vi "numberToString.vi"(8 "error in (no error)":errorcluster, 10 "Numeric":dbl, 11 "ScriptEvent in":refnum<class "ScriptEvent.lvclass">) -> (0 "error out":errorcluster, 2 "String":string, 3 "ScriptEvent out":refnum<class "ScriptEvent.lvclass">)   [LabVIEW 2009, in "Tools.lvlib" / "Scripting.lvlib" / "ScriptEvent.lvclass"]
uses:
  ScriptEvent.lvclass
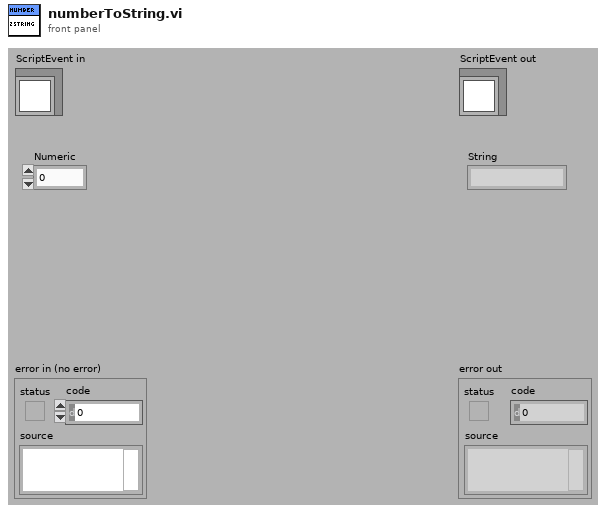
[diagram p1: front panel]
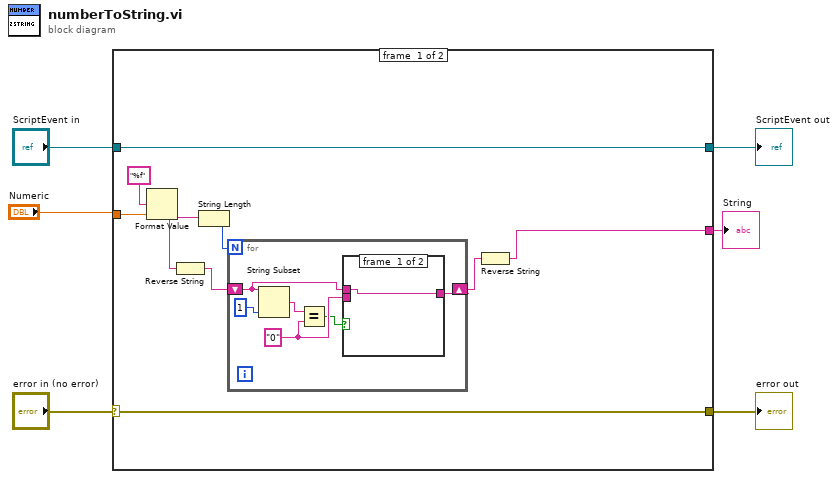
[diagram p0: block diagram]
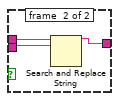
[diagram p2: hidden frame]
diagram:
  n1 = case shown="No Error" "error in (no error)" {
    selector: "error in (no error)" -> [w14 w27]
    tunnel: [w14 w27] -> w2
    tunnel: [w15 w26] -> w3
    tunnel: "ScriptEvent in" -> [w15 w26]
    tunnel: "Numeric" -> [w8 _]
    tunnel: [w7 _] -> w1
    frame #0 {
      n2 = Format Value(format string="%f", value (0)=w8) -> (output string=w9:string)  [unwired: 1 in]
      n3 = Reverse String(1:w9) -> (0:w12:string)
      n4 = String Length(string=w9) -> (length=w11:i32)
      n5 = for {
        N: w11 -> [_]
        shift-right: [w16] -> w10
        shift-left: w12 -> [w19]
        w18 = "0"
        n6 = String Subset(string=w19, length (rest)=1) -> (substring=w20:string)  [unwired: 1 in]
        n7 = Equal?(x=w20, y=w18) -> (x = y?=w17:bool)
        n8 = case shown="True" w17 {
          tunnel: w19 -> [w22 w25]
          tunnel: w18 -> [_ w23]
          tunnel: [w22 w24] -> w16
          frame #0 {
          }
          frame #1 {
            n9 = Search and Replace String(input string=w25, search string=w23) -> (result string=w24:string)  [unwired: 6 in, 3 out]
          }
        }
      }
      n10 = Reverse String(1:w10) -> (0:w7:string)
    }
    frame #1 {
    }
  }
  "error out" <- w2
  "ScriptEvent out" <- w3
  "String" <- w1
